vi "Configure Modulation (Frequency Shift Keying).vi"(0 "VISA resource name":refnum<visa-resource-name>, 1 "Enable FSK Modulation (T: Enable)":bool=TRUE, 5 "Channel (0: Channel 1)":u16(ring) items=["Channel 1", "Channel 2"], 9 "FSK Modulation Source (0: Internal)":u16(ring) items=["Internal", "External"], 11 "error in (no error)":errorcluster, 12 "Internal Rate (10.00 Hz)":dbl=10.0 format="%.2f", 13 "Hop Frequency (100.00 Hz)":dbl=100.0 format="%.2f") -> (4 "VISA resource name out":refnum<visa-resource-name>, 15 "error out":errorcluster)   [LabVIEW 2019, in "Tektronix AFG 3000 Series.lvlib"]
doc: "Configures and enables Frequency-Shift Keying (FSK) modulation. The function generator shifts its output frequency between two present values.\n\n<B> Note:</B>\n\nThe Pulse, Noise, and DC waveform functions are not valid for Configure Modulation (Frequency Shift Keying)."
uses:
  Tektronix AFG 3000 Series.lvlib
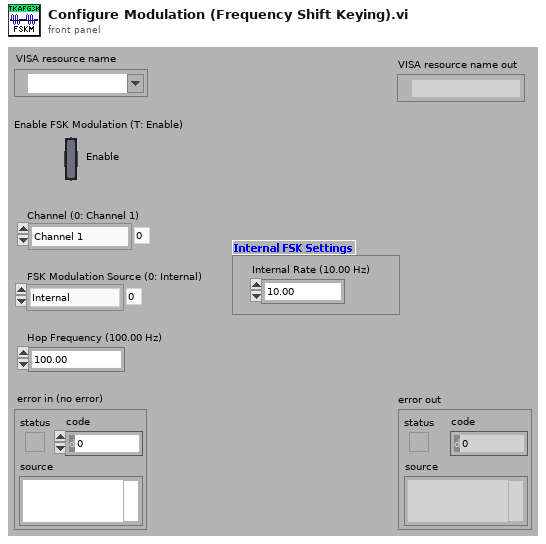
[diagram p1: front panel]
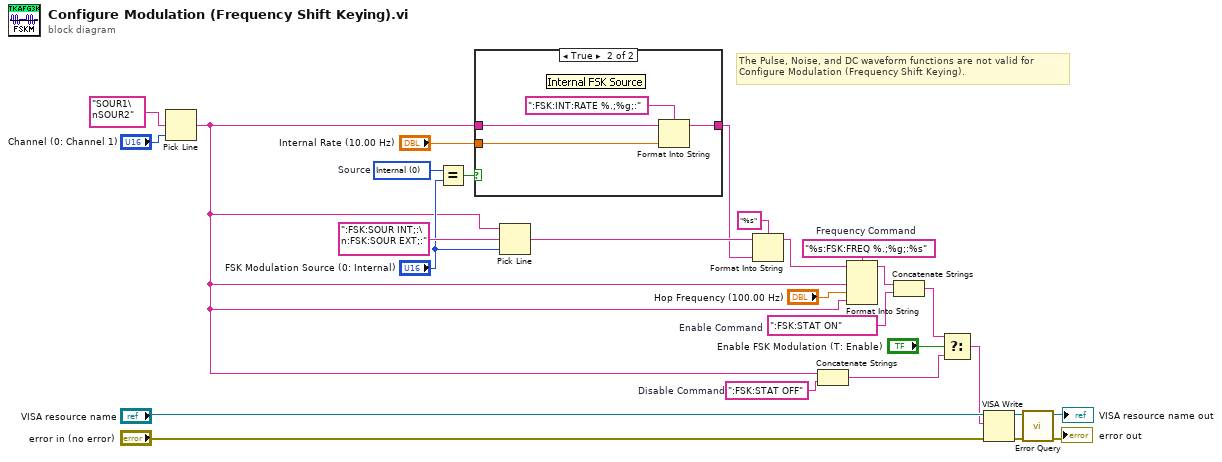
[diagram p0: block diagram]
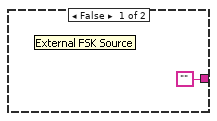
[diagram p2: hidden frame]
diagram:
  w19 = "%s:FSK:FREQ %.;%g;:%s"  # Frequency Command
  w20 = ":FSK:STAT ON"  # Enable Command
  w8 = u16 0 items=["Internal", "External"]  # Source
  w12 = ":FSK:STAT OFF"  # Disable Command
  # "The Pulse, Noise, and DC waveform functions are not valid for \nConfigure Modulation (Frequency Shift Keying)."
  n1 = Pick Line(multi-line string="SOUR1\nSOUR2" ("string (\"\")"), line index="Channel (0: Channel 1)") -> (output string=w2:string)  [unwired: 1 in]
  n2 = Equal?(x=w8, y="FSK Modulation Source (0: Internal)") -> (x = y?=w10:bool)
  n3 = case shown="True" w10 {
    tunnel: ["" w31] -> w5
    tunnel: w2 -> [_ w30]
    tunnel: "Internal Rate (10.00 Hz)" -> [_ w29]
    frame False {
    }
    frame True {
      n4 = Format Into String(format string=":FSK:INT:RATE %.;%g;:" ("initial string"), initial string=w30, w29) -> (resulting string=w31:string)  [unwired: 1 in, 1 out]
    }
  }
  n5 = Pick Line(string ("")=w2, multi-line string=":FSK:SOUR INT;:\n:FSK:SOUR EXT;:" ("string (\"\")"), line index="FSK Modulation Source (0: Internal)") -> (output string=w7:string)
  n6 = Format Into String(format string="%s", initial string=w7, w5) -> (resulting string=w4:string)  [unwired: 1 in, 1 out]
  n7 = Concatenate Strings(w2, w12) -> (w11:string)
  n8 = Format Into String(format string=w19, initial string=w4, w2, "Hop Frequency (100.00 Hz)", w2) -> (resulting string=w21:string)  [unwired: 1 in, 1 out]
  n9 = Concatenate Strings(w21, w20) -> (w13:string)
  n10 = Select(t=w13, s="Enable FSK Modulation (T: Enable)", f=w11) -> (s? t:f=w14:string)
  n11 = VISA Write(VISA resource name="VISA resource name", write buffer=w14, error in (no error)="error in (no error)") -> (VISA resource name out=w26:refnum<visa-resource-name>, error out=w25:errorcluster)  [unwired: 1 out]
  n12 = call "Error Query.vi"("error in (no error)"=w25, "VISA resource name"=w26) -> ("error out"=→"error out":errorcluster, "VISA resource name out"=→"VISA resource name out":refnum<visa-resource-name>)  [unwired: 6 in, 2 out]
